vi "(Depricated) Preview Syringe Pressure State.vi"(8 "error in (no error)":errorcluster, 9 "timeout in ms (0)":i32, 11 "cRIO Vacuum in":refnum<class "cRIO Vacuum.lvclass">) -> (0 "error out":errorcluster, 1 "Pressure (mBar)":dbl, 2 "Syringe Pressure State":T1, 3 "cRIO Vacuum out":refnum<class "cRIO Vacuum.lvclass">, 4 "timed out?":bool, 5 "d/dt":dbl, 6 "Raw Pressure":dbl)   [LabVIEW 2015]
uses:
  cRIO Vacuum.lvclass
  Controls/Vacuum State Enumerator.ctl
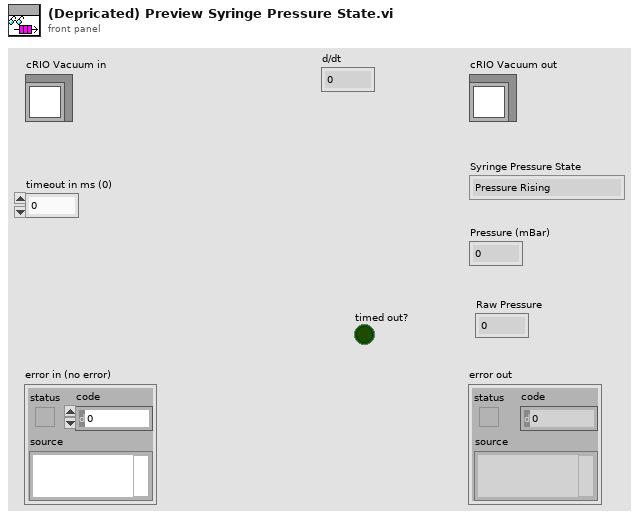
[diagram p1: front panel]
types:
  T1 = typedef "Vacuum State Enumerator.ctl" = enum16{"Pressure Rising", "Plateau", "Pressure Dropping", "Valley", "Low Valley", "Leak", "Unknown"}
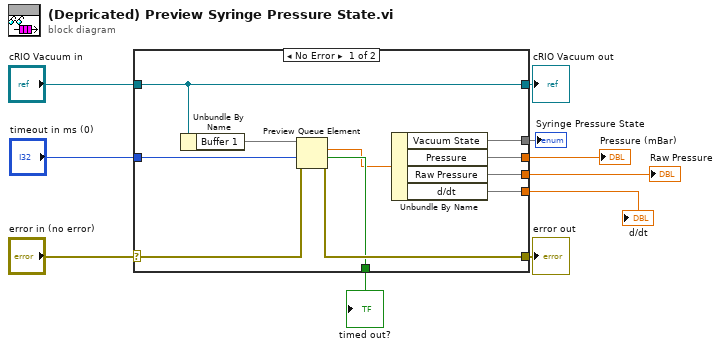
[diagram p0: block diagram]
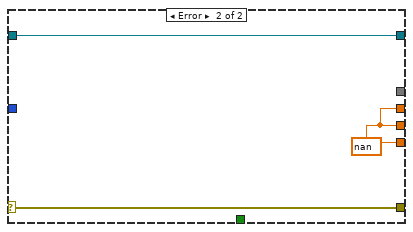
[diagram p2: hidden frame]
diagram:
  n1 = case shown="No Error" "error in (no error)" {
    selector: "error in (no error)" -> [w19 w23]
    tunnel: [w18 w23] -> w9
    tunnel: [w21 w24] -> w7
    tunnel: "cRIO Vacuum in" -> [w21 w24]
    tunnel: [w16 _] -> w6
    tunnel: "timeout in ms (0)" -> [w17 _]
    tunnel: [w15 w22] -> w4
    tunnel: [w14 _] -> w3
    tunnel: [w13 w22] -> w2
    tunnel: [w11 w22] -> w1
    frame No Error {
      n2 = Unbundle By Name(w21) -> ("Buffer 1"=w20)
      n3 = Preview Queue Element(queue=w20, timeout in ms (-1)=w17, error in (no error)=w19) -> (element=w12:dbl, timed out?=w14:bool, error out=w18:errorcluster)  [unwired: 1 out]
      n4 = Unbundle By Name(w12) -> ("Vacuum State"=w16, "Pressure"=w15, "Raw Pressure"=w13, "d/dt"=w11)
    }
    frame Error {
      w22 = nan ("Pressure")
    }
  }
  "error out" <- w9
  "cRIO Vacuum out" <- w7
  "Syringe Pressure State" <- w6
  "Pressure (mBar)" <- w4
  "timed out?" <- w3
  "Raw Pressure" <- w2
  "d/dt" <- w1
